vi "testVI.vi"() -> ()   [LabVIEW 2010]
uses:
  types/testCtl.ctl
  <vilib>/Utility/miscctls.llb/LVStringsAndValuesArrayTypeDef.ctl
panel:
  out "Colors [4]":cluster{u32, u32}[](array[cluster])
  out "Strings [4]":string[](array[string])
  out "OK Button":bool
  out "Strings And Values []":T1
  out "Digital Display.Text":string
  in  "Cluster":T2
  out "Ring Text.Text":string
  out "Ring 2":u16(ring) items=["start", "end", "on", "off", "elf"]
  in  "Ring":u16(ring)
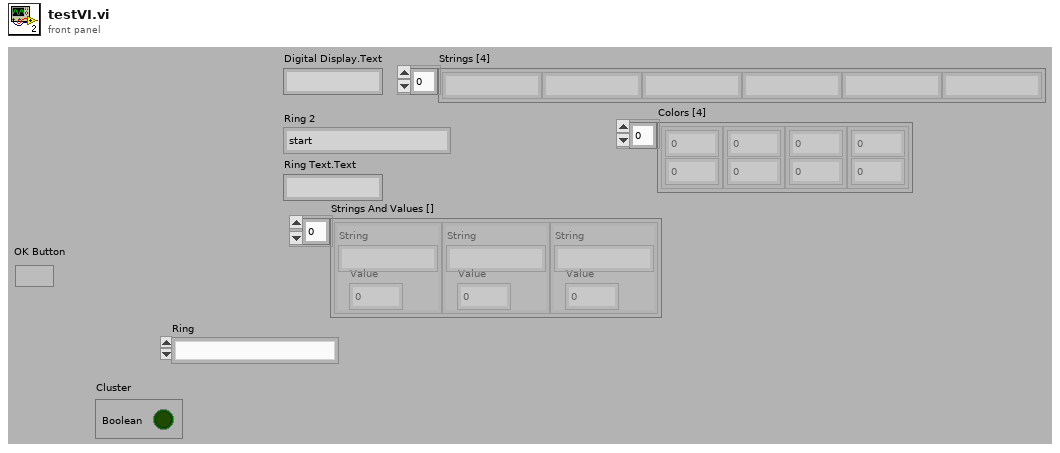
[diagram p1: front panel]
types:
  T1 = typedef "LVStringsAndValuesArrayTypeDef.ctl" = cluster{"String":string, "Value":ext}[]
  T2 = typedef "testCtl.ctl" = cluster{"Boolean":bool, "String":string}
  T3 = typedef "LVStringsAndValuesArrayTypeDef.ctl" = cluster{"String":string, "Value":u16}[]
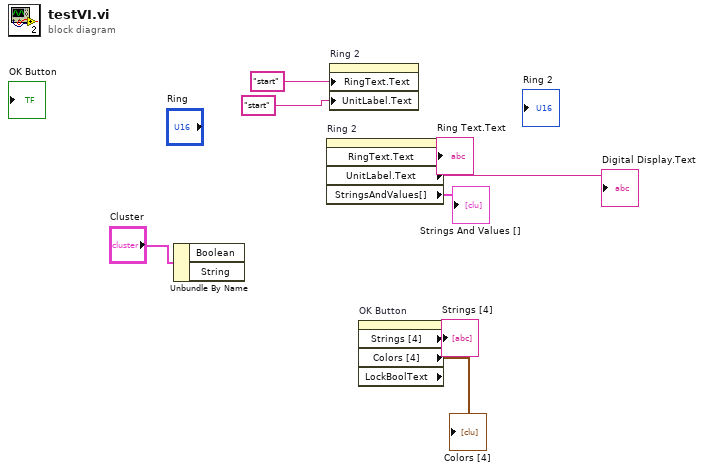
[diagram p0: block diagram]
diagram:
  n1 = Unbundle By Name("Cluster") -> ()  [unwired: 2 out]
  n2 = property on="Ring 2" class="Ring (strict)"() -> ("RingText.Text"=→"Ring Text.Text":string, "UnitLabel.Text"=→"Digital Display.Text":string, "StringsAndValues[]"=→"Strings And Values []":T3)  [unwired: 2 in, 2 out]
  n3 = property on="Ring 2" class="Ring (strict)"("RingText.Text"="start" ("Ring Text.Text"), "UnitLabel.Text"="start" ("Digital Display.Text")) -> ()  [unwired: 2 in, 2 out]
  n4 = property on="OK Button" class="Bool (strict)" props=["Strings [4]", "Colors [4]", "LockBoolText"]() -> ("Strings [4]"=→"Strings [4]":string[], "Colors [4]"=→"Colors [4]":cluster{u32, u32}[])  [unwired: 2 in, 3 out]
